vi "comms_BT_Read_File.vi"(8 "error in":errorcluster, 9 "filename":string="temp.dat", 10 "file path (use dialog)":path, 11 "connection ID":refnum<k31>) -> (0 "error out":errorcluster, 3 "connection ID out":refnum<k31>)   [LabVIEW 2016]
panel:
  in  "Stop Button":bool
  out "Total Packets":dbl
  out "Packet":dbl
  out "Transfer Speed (Bytes/S)":i64
  out "Elapsed Time (s)":i64
  out "data packet":string
  out "Error?":bool
  out "filesize":string
  out "File Size (Bytes)":i64
  out "Transfer Progress":dbl(slide) scale=0.0..100.0
  # "Receiving File..."
  # "of"
  # "s"
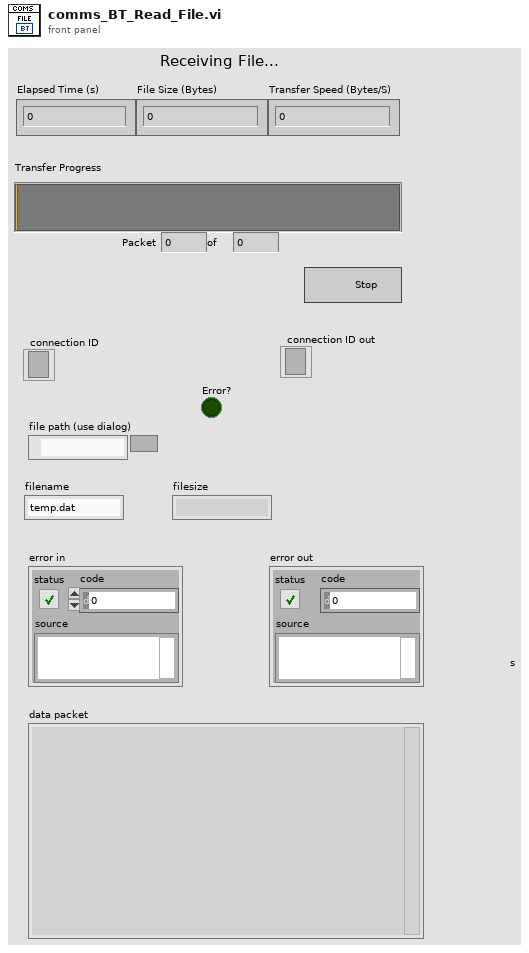
[diagram p1: front panel]
types:
  T1 = enum16{"open", "replace", "create", "open or create", "replace or create", "replace or create with confirmation"}
  T2 = enum16{"Standard", "Buffered", "CRLF", "Immediate"}
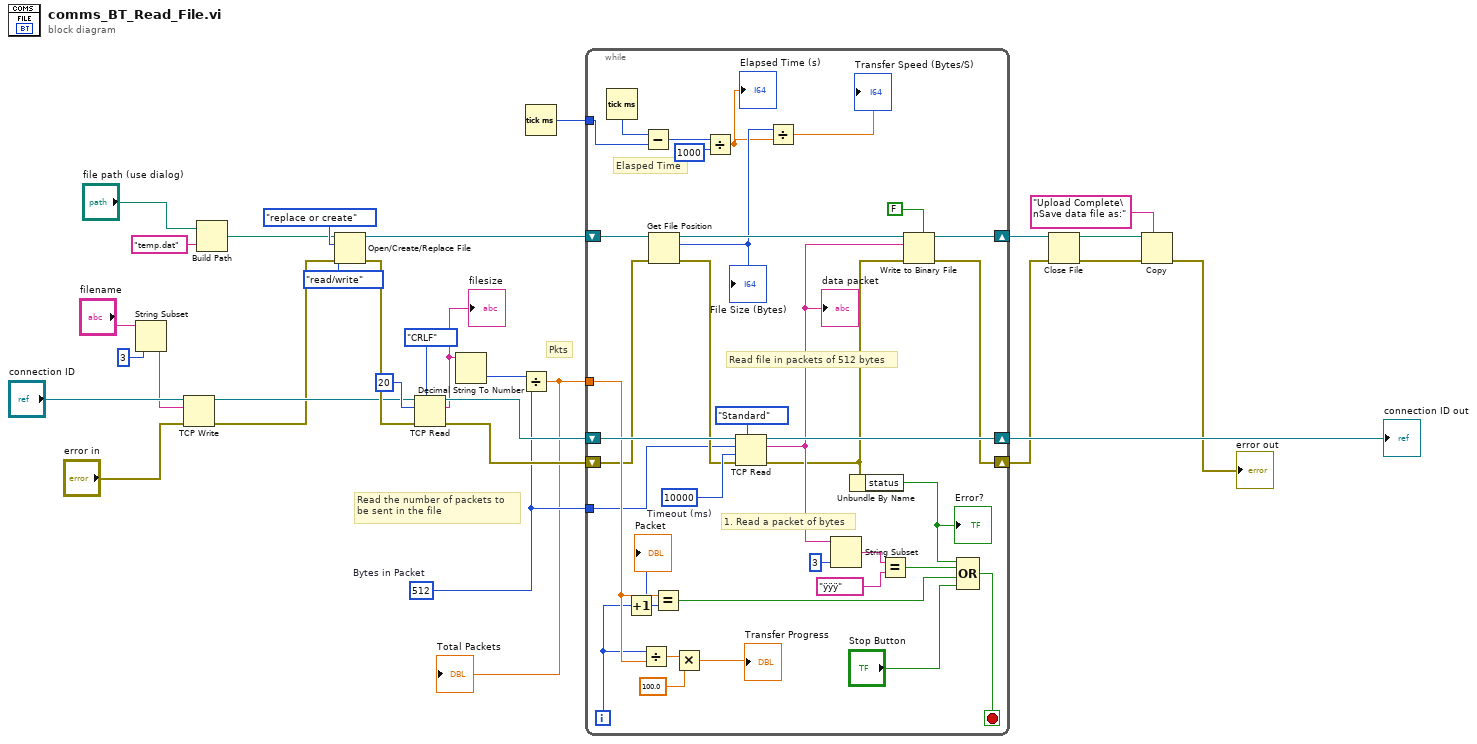
[diagram p0: block diagram]
diagram:
  w3 = 512  # Bytes in Packet
  # "Pkts"
  # "Read the number of packets to\nbe sent in the file"
  n1 = String Subset(string="filename", length (rest)=3 ("length (rest)")) -> (substring=w8:string)  [unwired: 1 in]
  n2 = TCP Write(connection ID="connection ID", data in=w8, error in (no error)="error in") -> (connection ID out=w10:refnum<k31>, error out=w5:errorcluster)  [unwired: 1 in, 1 out]
  n3 = Build Path(base path="file path (use dialog)", name or relative path="temp.dat") -> (appended path=w17:path)
  n4 = Open/Create/Replace File(file path (use dialog)=w17, error in=w5, operation (0:open)=T1."replace or create", access (0:read/write)=enum16{"read/write", "read-only", "write-only"}."read/write") -> (refnum out=w21:refnum<file>, error out=w23:errorcluster)  [unwired: 2 in, 1 out]
  n5 = TCP Read(connection ID=w10, bytes to read=20, error in (no error)=w23, 7:T2."CRLF" ("mode (standard)")) -> (connection ID out=w30:refnum<k31>, data out=w28:string, error out=w29:errorcluster)  [unwired: 1 in]
  "filesize" <- w28
  n6 = Decimal String To Number(string=w28) -> (number=w4:i32)  [unwired: 2 in, 1 out]
  n7 = Divide(x=w4, y=w3) -> (x/y=w1:dbl)
  "Total Packets" <- w1
  n8 = Tick Count (ms)() -> (millisecond timer value=w2:u32)
  n9 = while {
    shift-right: [w57] -> w19
    shift-left: w29 -> [w48]
    tunnel: w1 -> [w53]
    shift-right: [w56] -> w20
    shift-left: w21 -> [w50]
    shift-right: [w62] -> w25
    shift-left: w30 -> [w65]
    tunnel: w3 -> [w46]
    tunnel: w2 -> [w42]
    i -> [w52]
    stop <- w32 stop-if-true
    w63 = 10000  # Timeout (ms)
    # "Elasped Time"
    # "Read file in packets of 512 bytes"
    # "1. Read a packet of bytes"
    n10 = Tick Count (ms)() -> (millisecond timer value=w43:u32)
    n11 = Increment(x=w52) -> (x+1=w38:i32)
    "Packet" <- w38
    n12 = Divide(x=w52, y=w53) -> (x/y=w55:dbl)
    n13 = Subtract(x=w43, y=w42) -> (x-y=w40:u32)
    n14 = Get File Position(4:w48, 7:w50) -> (0:w47:errorcluster, 2:w41:i64, 3:w49:refnum<file>)
    "File Size (Bytes)" <- w41
    n15 = Equal?(x=w53, y=w38) -> (x = y?=w33:bool)
    n16 = Multiply(x=w55, y=100.0) -> (x*y=→"Transfer Progress":dbl)
    n17 = Divide(x=w40, y=1000 ("bytes to read")) -> (x/y=w36:dbl)
    "Elapsed Time (s)" <- w36
    n18 = TCP Read(connection ID=w65, bytes to read=w46, error in (no error)=w47, 7:T2."Standard" ("mode (standard)"), 9:w63) -> (connection ID out=w62:refnum<k31>, data out=w58:string, error out=w45:errorcluster)
    "data packet" <- w58
    n19 = Divide(x=w41, y=w36) -> (x/y=→"Transfer Speed (Bytes/S)":dbl)
    n20 = String Subset(string=w58, length (rest)=3 ("length (rest)")) -> (substring=w60:string)  [unwired: 1 in]
    n21 = Unbundle By Name(w45) -> ("status"=w35:bool)
    "Error?" <- w35
    n22 = Equal?(x=w60, y="ÿÿÿ") -> (x = y?=w34:bool)
    n23 = Write to Binary File(file (use dialog)=w49, data=w58, error in=w45, 5:FALSE ("prepend array or string size? (T)")) -> (refnum out=w56:refnum<file>, error out=w57:errorcluster)  [unwired: 2 in, 1 out]
    n24 = Compound Arithmetic op=OR(w35, w34, w33, "Stop Button") -> (w32:bool)
  }
  "connection ID out" <- w25
  n25 = Close File(refnum=w20, error in=w19) -> (path=w15:path, error out=w13:errorcluster)
  n26 = Copy(7:"Upload Complete\nSave data file as:" ("prompt (Choose or enter target path for copy)"), 8:w13, 11:w15) -> (0:→"error out":errorcluster)  [unwired: 2 in, 2 out]
